vi "Measure - NI 9263.vi"(8 "error in":errorcluster) -> (0 "error out":errorcluster={"status"=TRUE, "code"=-200088, "source"="Property Node DAQmx Timing (arg 1) in WaveformBufferGeneration_(multi).vi->Measure - NI 9263.vi <append>\n"})   [LabVIEW 2011]
doc: "I. Description:\nThis example demonstrates how to output a continuous periodic waveform using an internal sample clock.\n\nII. Instructions for Running:\n1. Select the Physical Channel to correspond to where your signal is output on the DAQ device.\n2. Enter the Minimum and Maximum Voltage Ranges\n3. Specify the Desired Frequency of the output Waveform\n4. Enter the Waveform Information. See the documentation of the Waveform Buffer Generation SubVI for information on each parameter.\n\nIII. Block Diagram Steps:\n1. Create an Analog Output Voltage channel.\n2. Call the DAQmx Timing (Use Waveform) VI which sets the sample clock rate based on the input waveform parameters, and set the sample mode to Continuous.\n3. Write the waveform to the output buffer.\n4. Call the Start VI.\n5. Loop continuously until the user presses the Stop button. Check for errors every 100 ms using the Is Task Done? VI\n6. Clear the Task\n7. Use the popup dialog box to display an error or warning if any.\n\nIV. I/O Connections Overview:\nMake sure your signal output terminal matches the Physical Channel I/O Control. For further connection information, refer to your hardware reference manual."
uses:
  <vilib>/DAQmx/write.llb/DAQmx Write (Analog 1D Wfm NChan NSamp).vi
  <vilib>/DAQmx/configure/timing.llb/DAQmx Timing (Use Waveform).vi
  <vilib>/DAQmx/miscellaneous.llb/DAQmx Fill In Error Info.vi
panel:
  out "Waveform Chart":waveform(dbl)[](graph)
  in  "Amplitude":dbl=2.0
  in  "Cycles per Buffer":i32=10 caption="Cycles"
  in  "Waveform Type":T1(ring)
  in  "Samples per Buffer":dbl=200.0 caption="Samples"
  in  "Update":bool
  in  "Exit":bool
  out "Resulting Frequency":dbl format="%.2f"
  in  "Desired Frequency":dbl=500.0 format="%.2f"
  # "Waveform Information"
  # "Timing Parameters"
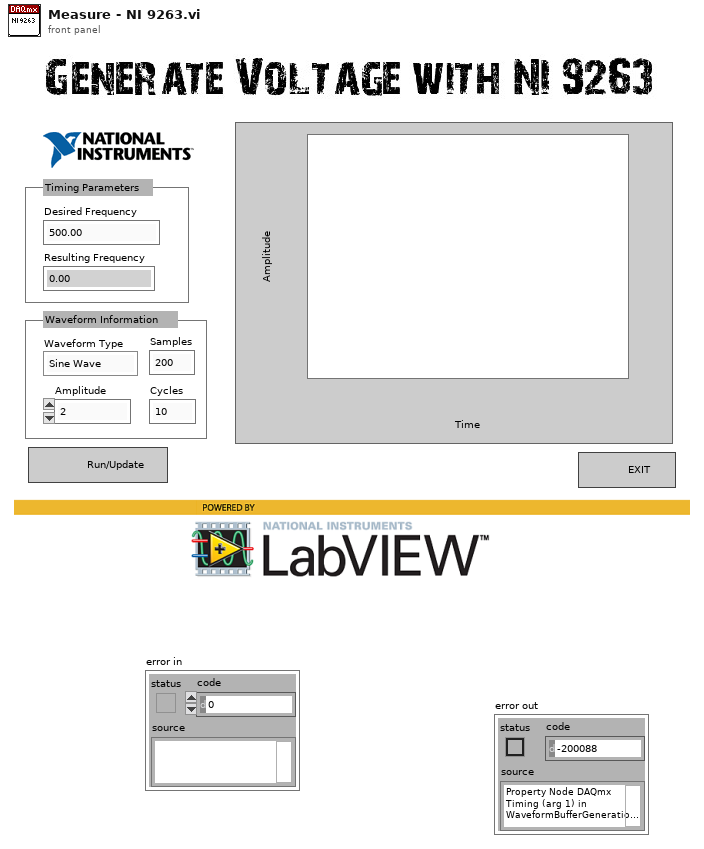
[diagram p1: front panel]
types:
  T1 = enum16{"Sine Wave", "Triangle Wave", "Square Wave", "Sawtooth Wave"}
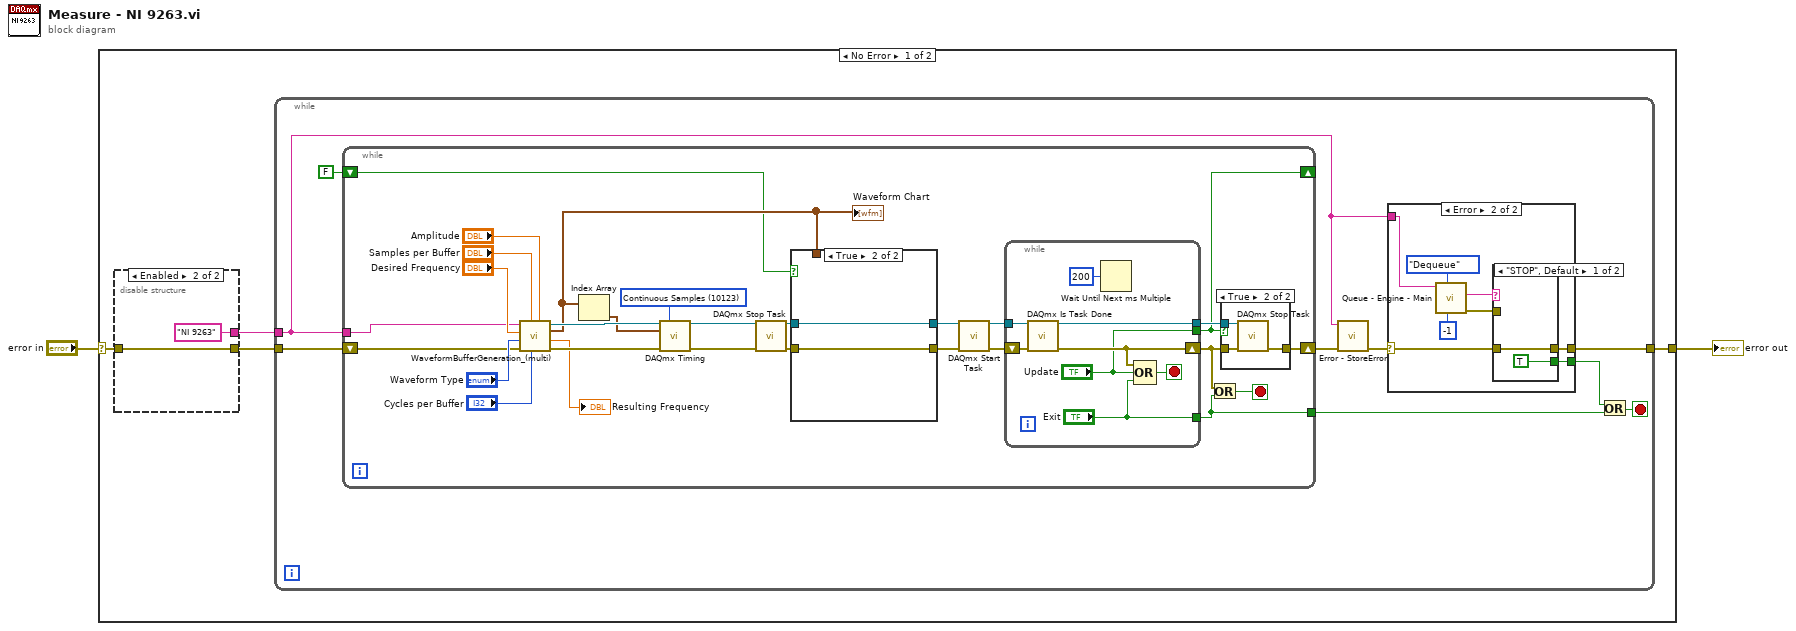
[diagram p0: block diagram]
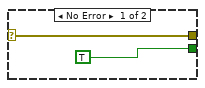
[diagram p2: hidden frame]
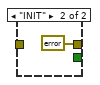
[diagram p3: hidden frame]
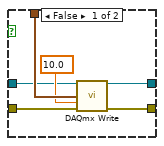
[diagram p4: hidden frame]
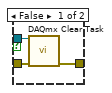
[diagram p5: hidden frame]
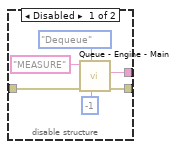
[diagram p6: hidden frame]
diagram:
  n1 = case shown="No Error" "error in" {
    selector: "error in" -> [w6 w87]
    tunnel: [w3 w87] -> w2
    frame No Error {
      n2 = disable-structure shown="Enabled" {
        disable-tunnel: w6 -> [w84 w86]
        disable-tunnel: [w83 w86] -> w5
        disable-tunnel: [w82 "NI 9263" ("Data Out")] -> w4
        frame Disabled {
          n3 = call "Queue - Engine - Main.vi"("timeout in ms (-1)"=-1, "Operation"=enum16{"Enqueue", "Dequeue", "Flush", "Release"}."Dequeue", "error in"=w84, "Queue Name In"="MEASURE") -> ("error out"=w83:errorcluster, "Data Out"=w82:string)  [unwired: 5 in, 1 out]
        }
        frame Enabled {
        }
      }
      n4 = while {
        tunnel: w5 -> [w15]
        tunnel: w4 -> [w10]
        tunnel: [w11] -> w3
        stop <- w7 stop-if-true
        n5 = while {
          shift-right: [w43] -> w13
          shift-left: w15 -> [w31]
          tunnel: w10 -> [w30]
          shift-right: [w33] -> _
          shift-left: FALSE ("Update") -> [w32]
          tunnel: [w29] -> w8
          stop <- w40 stop-if-true
          w39 = 10123 items=["Finite Samples"=10178, "Continuous Samples"=10123] ("sample mode")
          n6 = call "WaveformBufferGeneration_(multi).vi"("Amplitude"="Amplitude", "Cycles per Buffer"="Cycles per Buffer", "Samples per Buffer"="Samples per Buffer", "error in (no error)"=w31, "Waveform Type"="Waveform Type", "Desired Frequency"="Desired Frequency", "task/channels in"=w30) -> ("error out"=w50:errorcluster, "Resulting Frequency"=→"Resulting Frequency":dbl, "Waveform"=w38:waveform(dbl)[], "task out"=w51:refnum<k21>)  [unwired: 1 out]
          "Waveform Chart" <- w38
          n7 = Index Array(array=w38) -> (element=w44:waveform(dbl))  [unwired: 1 in]
          n8 = call-poly <vilib>:"DAQmx Timing.vi"("task/channels in"=w51, "sample mode"=w39, "waveform"=w44, "error in"=w50) -> ("task out"=w35:refnum<k21>, "error out"=w37:errorcluster)  [unwired: 10 in]
          n9 = call <vilib>:"DAQmx Stop Task.vi"("task/channels in"=w35, "error in"=w37) -> ("task out"=w34:refnum<k21>, "error out"=w36:errorcluster)  [unwired: 12 in]
          n10 = case shown="True" w32 {
            tunnel: [w62 w63] -> w56
            tunnel: [w61 w64] -> w55
            tunnel: w38 -> [w60 _]
            tunnel: w36 -> [w58 w64]
            tunnel: w34 -> [w57 w63]
            frame False {
              n11 = call-poly <vilib>:"DAQmx Write.vi"("task/channels in"=w57, "data"=w60, "timeout"=10.0 ("Wirite Timeout"), "error in"=w58) -> ("task out"=w62:refnum<k21>, "error out"=w61:errorcluster)  [unwired: 9 in, 1 out]
            }
            frame True {
            }
          }
          n12 = call <vilib>:"DAQmx Start Task.vi"("task/channels in"=w56, "error in"=w55) -> ("task out"=w53:refnum<k21>, "error out"=w54:errorcluster)  [unwired: 12 in]
          n13 = while {
            tunnel: w53 -> [w78]
            tunnel: [w77] -> w52
            tunnel: ["Exit"] -> w29
            shift-right: [w74] -> w41
            shift-left: w54 -> [w76]
            tunnel: ["Update"] -> w33
            stop <- w72 stop-if-true
            n14 = call <vilib>:"DAQmx Is Task Done.vi"("task/channels in"=w78, "error in"=w76) -> ("task out"=w77:refnum<k21>, "error out"=w74:errorcluster)  [unwired: 11 in, 1 out]
            n15 = Wait Until Next ms Multiple(millisecond multiple=u32 200) -> ()  [unwired: 1 out]
            n16 = Compound Arithmetic op=OR(w74, "Update", "Exit") -> (w72:bool)
          }
          n17 = Or(x=w41, y=w29) -> (x .or. y?=w40:bool)
          n18 = case shown="True" w33 {
            tunnel: w52 -> [w67 w70]
            tunnel: [w66 w68] -> w43
            tunnel: w41 -> [w65 w69]
            frame False {
              n19 = call <vilib>:"DAQmx Clear Task.vi"("task in"=w67, "error in"=w65) -> ("error out"=w66:errorcluster)  [unwired: 13 in]
            }
            frame True {
              n20 = call <vilib>:"DAQmx Stop Task.vi"("task/channels in"=w70, "error in"=w69) -> ("error out"=w68:errorcluster)  [unwired: 12 in, 1 out]
            }
          }
        }
        n21 = call "Error - StoreError.vi"("Error In"=w13, "Error Source In"=w10) -> ("Error Out"=w12:errorcluster)  [unwired: 8 in, 1 out]
        n22 = case shown="Error" w12 {
          selector: w12 -> [w17 w18]
          tunnel: [w17 w20] -> w11
          tunnel: [TRUE w19] -> w9
          tunnel: w10 -> [_ w23]
          frame No Error {
          }
          frame Error {
            n23 = call "Queue - Engine - Main.vi"("timeout in ms (-1)"=-1, "Operation"=enum16{"Enqueue", "Dequeue", "Flush", "Release"}."Dequeue", "Queue Name In"=w23) -> ("error out"=w22:errorcluster, "Data Out"=w21:string)  [unwired: 6 in, 1 out]
            n24 = case shown="\"STOP\", Default" w21 {
              tunnel: w22 -> [_ _]
              tunnel: [w26 errorcluster {"status"=FALSE, "code"=0, "source"=""} ("error out")] -> w20
              tunnel: [TRUE _] -> w19
              tunnel: w18 -> [w26 _]
              frame "STOP", Default {
              }
              frame "INIT" {
              }
            }
          }
        }
        n25 = Or(x=w9, y=w8) -> (x .or. y?=w7:bool)
      }
    }
    frame Error {
    }
  }
  "error out" <- w2
